vi "SiosIfmGetDeviceInfoFirmwareVersion.vi"(1 "devNumber":i32) -> (0 "Ausgabe-Parameter":string)   [LabVIEW 2009]
uses:
  siosifm.dll
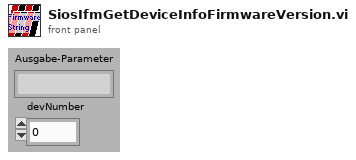
[diagram p1: front panel]
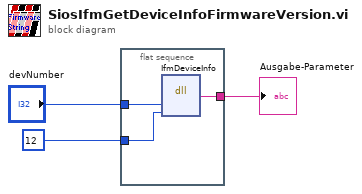
[diagram p0: block diagram]
diagram:
  n1 = flat-sequence {
    tunnel: [w6] -> w3
    tunnel: "devNumber" -> [w5]
    tunnel: 12 ("requestedInfo") -> [w4]
    frame #0 {
      n2 = dll-call lib="C:/WORK/Artem/RE-10/SIOS_IfmDLL/siosifm.dll" fn="IfmDeviceInfo"("devNumber"=w5, "requestedInfo"=w4) -> (w6:string)  [unwired: 5 in, 2 out]
    }
  }
  "Ausgabe-Parameter" <- w3
